vi "Test_dout0 to din0.vi"(6 "VISA resource name":refnum<visa-resource-name>, 7 "Passed so far?":bool, 8 "error in (no error)":errorcluster, 10 "Dout0 ON (y)":bool=TRUE, 11 "Slot":T1) -> (0 "error out":errorcluster, 3 "Din APx ON?":bool, 4 "VISA resource name out":refnum<visa-resource-name>, 5 "Passed?":bool)   [LabVIEW 2024]
uses:
  AP slots to test.ctl
  <vilib>/Instr/_visa.llb/VISA Configure Serial Port (Instr).vi
panel:
  out "read buffer 2":string
  out "Din AP2 ON?":bool
  out "read buffer":string
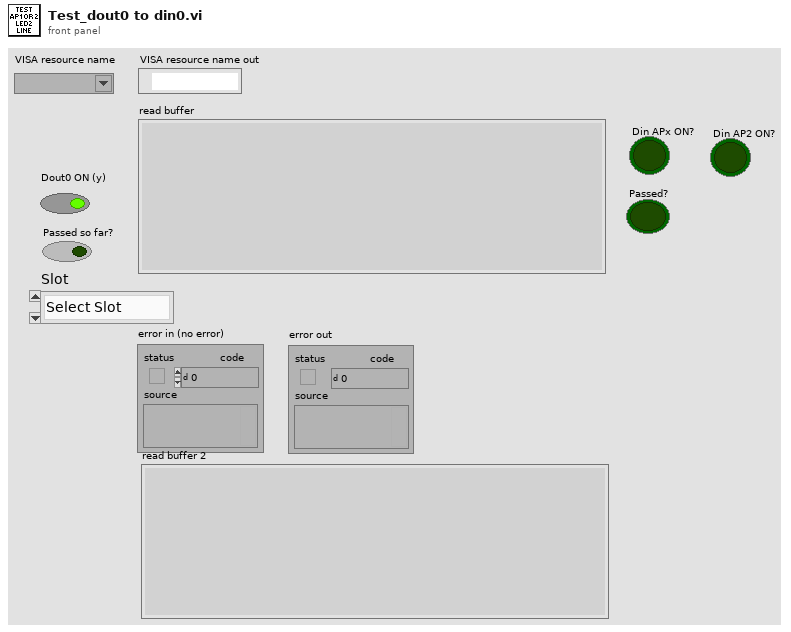
[diagram p1: front panel]
types:
  T1 = typedef "AP slots to test.ctl" = enum16{"Select Slot", "AP1", "AP2", "AP1 and AP2"}
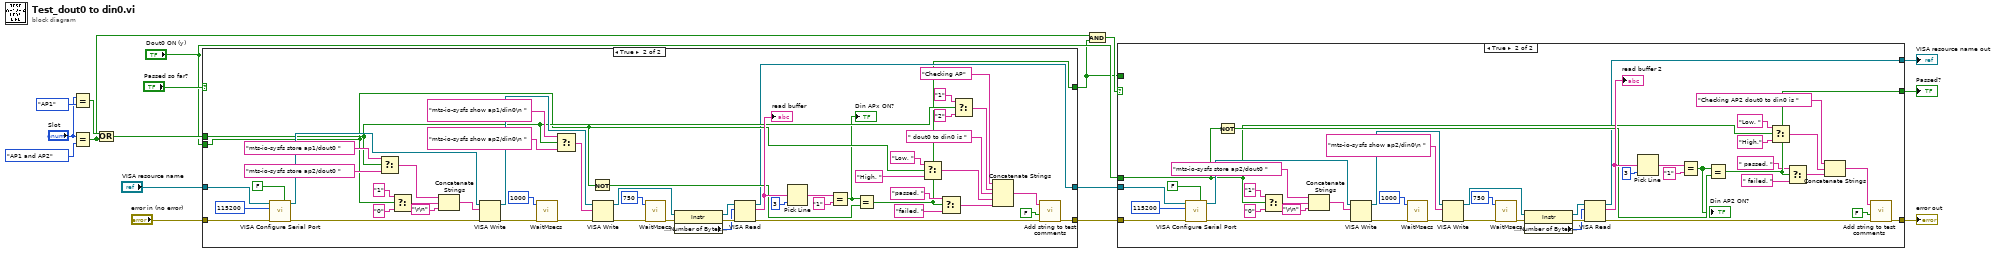
[diagram p0: block diagram]
diagram:
  n1 = Equal?(x="Slot", y=AP_slots_to_test."AP1") -> (x = y?=w13:bool)
  n2 = Equal?(x="Slot", y=AP_slots_to_test."AP1 and AP2") -> (x = y?=w3:bool)
  n3 = Or(x=w13, y=w3) -> (x .or. y?=w12:bool)
  n4 = case shown="True" "Passed so far?" {
    selector: "Passed so far?" -> [w18 _]
    tunnel: [w20 w27] -> w8
    tunnel: "Dout0 ON (y)" -> [_ w36]
    tunnel: w12 -> [_ w37]
    tunnel: "error in (no error)" -> [w20 w42]
    tunnel: "VISA resource name" -> [w19 w25]
    tunnel: [w19 w24] -> w9
    tunnel: [w18 w21] -> w1
    frame False {
    }
    frame True {
      n5 = call-poly "VISA Configure Serial Port"("VISA resource name"=w25, "Enable Termination\nChar (T)"=FALSE ("Enable Termination\nChar (T)"), "baud rate (9600)"=u32 115200, "error in (no error)"=w42) -> ("VISA resource name out"=w71:refnum<visa-resource-name>, "error out"=w70:errorcluster)  [unwired: 10 in]
      n6 = Select(t="mts-io-sysfs store ap1/dout0 ", s=w37, f="mts-io-sysfs store ap2/dout0 ") -> (s? t:f=w49:string)
      n7 = Select(t="1", s=w36, f="0") -> (s? t:f=w46:string)
      n8 = Concatenate Strings(w49, w46, "\r\n") -> (w45:string)
      n9 = VISA Write(VISA resource name=w71, write buffer=w45, error in (no error)=w70) -> (VISA resource name out=w58:refnum<visa-resource-name>, error out=w63:errorcluster)  [unwired: 1 out]
      n10 = call "WaitMsecs.vi"("error in (no error)"=w63, "Wait Msecs"=u32 1000) -> ("error out"=w56:errorcluster)  [unwired: 9 in]
      n11 = Select(t="mts-io-sysfs show ap1/din0\n ", s=w37, f="mts-io-sysfs show ap2/din0\n ") -> (s? t:f=w57:string)
      n12 = Not(x=w36) -> (.not. x?=w43:bool)
      n13 = VISA Write(VISA resource name=w58, write buffer=w57, error in (no error)=w56) -> (VISA resource name out=w55:refnum<visa-resource-name>, error out=w53:errorcluster)  [unwired: 1 out]
      n14 = call "WaitMsecs.vi"("error in (no error)"=w53, "Wait Msecs"=u32 750) -> ("error out"=w52:errorcluster)  [unwired: 9 in]
      n15 = property class="Instr"(reference=w55, error in=w52) -> (reference out=w68:refnum<visa-resource-name>, error out=w67:errorcluster, "Serial Settings:Number of Bytes at Serial Port"=w66:u32)
      n16 = VISA Read(VISA resource name=w68, byte count=w66, error in (no error)=w67) -> (VISA resource name out=w24:refnum<visa-resource-name>, read buffer=w62:string, error out=w23:errorcluster)  [unwired: 1 out]
      "read buffer" <- w62
      n17 = Pick Line(multi-line string=w62, line index=3) -> (output string=w51:string)  [unwired: 1 in]
      n18 = Equal?(x=w51, y="1") -> (x = y?=w22:bool)
      "Din APx ON?" <- w22
      n19 = Equal?(x=w22, y=w43) -> (x = y?=w21:bool)
      n20 = Select(t="Low, ", s=w36, f="High, ") -> (s? t:f=w32:string)
      n21 = Select(t="passed. ", s=w21, f="failed. ") -> (s? t:f=w29:string)
      n22 = Select(t="1", s=w37, f="2") -> (s? t:f=w38:string)
      n23 = Concatenate Strings("Checking AP" ("string"), w38, " dout0 to din0 is " ("string"), w32, w29) -> (w28:string)
      n24 = call "Add string to test comments.vi"("error in (no error)"=w23, "New Section (y)?"=FALSE, "Comments"=w28) -> ("error out"=w27:errorcluster)  [unwired: 7 in, 1 out]
    }
  }
  n25 = And(x=w3, y=w1) -> (x .and. y?=w2:bool)
  n26 = case shown="True" w2 {
    tunnel: [w74 w88] -> w6
    tunnel: [w76 w83] -> w7
    tunnel: "Dout0 ON (y)" -> [_ w92]
    tunnel: w8 -> [w76 w94]
    tunnel: w9 -> [w75 w81]
    tunnel: [w75 w80] -> w5
    tunnel: w1 -> [w74 _]
    frame False {
    }
    frame True {
      n27 = call-poly "VISA Configure Serial Port"("VISA resource name"=w81, "Enable Termination\nChar (T)"=FALSE ("Enable Termination\nChar (T)"), "baud rate (9600)"=u32 115200, "error in (no error)"=w94) -> ("VISA resource name out"=w118:refnum<visa-resource-name>, "error out"=w117:errorcluster)  [unwired: 10 in]
      n28 = Not(x=w92) -> (.not. x?=w96:bool)
      n29 = Select(t="1", s=w92, f="0") -> (s? t:f=w99:string)
      n30 = Concatenate Strings("mts-io-sysfs store ap2/dout0 ", w99, "\r\n") -> (w98:string)
      n31 = VISA Write(VISA resource name=w118, write buffer=w98, error in (no error)=w117) -> (VISA resource name out=w109:refnum<visa-resource-name>, error out=w112:errorcluster)  [unwired: 1 out]
      n32 = call "WaitMsecs.vi"("error in (no error)"=w112, "Wait Msecs"=u32 1000) -> ("error out"=w108:errorcluster)  [unwired: 9 in]
      n33 = VISA Write(VISA resource name=w109, write buffer="mts-io-sysfs show ap2/din0\n ", error in (no error)=w108) -> (VISA resource name out=w107:refnum<visa-resource-name>, error out=w105:errorcluster)  [unwired: 1 out]
      n34 = call "WaitMsecs.vi"("error in (no error)"=w105, "Wait Msecs"=u32 750) -> ("error out"=w104:errorcluster)  [unwired: 9 in]
      n35 = property class="Instr"(reference=w107, error in=w104) -> (reference out=w115:refnum<visa-resource-name>, error out=w114:errorcluster, "Serial Settings:Number of Bytes at Serial Port"=w113:u32)
      n36 = VISA Read(VISA resource name=w115, byte count=w113, error in (no error)=w114) -> (VISA resource name out=w80:refnum<visa-resource-name>, read buffer=w111:string, error out=w79:errorcluster)  [unwired: 1 out]
      "read buffer 2" <- w111
      n37 = Pick Line(multi-line string=w111, line index=3) -> (output string=w103:string)  [unwired: 1 in]
      n38 = Equal?(x=w103, y="1") -> (x = y?=w95:bool)
      "Din AP2 ON?" <- w95
      n39 = Equal?(x=w95, y=w96) -> (x = y?=w88:bool)
      n40 = Select(t="Low, ", s=w92, f="High,") -> (s? t:f=w89:string)
      n41 = Select(t=" passed. ", s=w88, f=" failed. ") -> (s? t:f=w85:string)
      n42 = Concatenate Strings("Checking AP2 dout0 to din0 is " ("string"), w89, w85) -> (w84:string)
      n43 = call "Add string to test comments.vi"("error in (no error)"=w79, "New Section (y)?"=FALSE, "Comments"=w84) -> ("error out"=w83:errorcluster)  [unwired: 7 in, 1 out]
    }
  }
  "Passed?" <- w6
  "error out" <- w7
  "VISA resource name out" <- w5
